vi "Globals.vi"() -> ()   [LabVIEW 2018]
panel:
  in  "Sensor 2":bool
  in  "Sensor 1":bool
  out "ACK":bool
  out "HB":bool
  in  "Pump State":bool
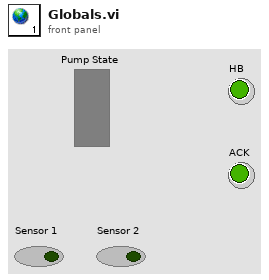
[diagram p1: front panel]
diagram:
